vi "Build-temperature-regression.vi"(8 "error in (no error)":errorcluster, 9 "Storage params in":refnum<data-value>, 10 "Acquis. params in":refnum<data-value>, 11 "Temperature params in":refnum<data-value>) -> (0 "error out":errorcluster, 1 "Storage params":refnum<data-value>, 2 "Acquis. params":refnum<data-value>, 3 "Temperature params":refnum<data-value>)   [LabVIEW 2013, in "CameraVision.lvlib" / "CV-Temperature.lvclass"]
uses:
  CV-Temperature.lvclass
  Acquisition/CV-Acquisition.lvclass
  Storage/CV-Storage.lvclass
  Storage/CV-Storage.lvclass/CV-Storage.ctl
  CV-Temperature.lvclass/CV-Temperature.ctl
  Acquisition/CV-Acquisition.lvclass/CV-Acquisition.ctl
  UI/Module-states.ctl
  Write Temperature status.vi
  Write TemperatureFieldRegression.vi
  Acquisition/Read Exposure time camera 1.vi
  Acquisition/Read Exposure time camera 2.vi
  Read Temperature field.vi
  Read Ratio correction factor.vi
  Read Regression file relative path.vi
  Storage/Read Base path.vi
  <vilib>/Utility/file.llb/Read From Spreadsheet File (DBL).vi
  UI/CV-UI.lvclass
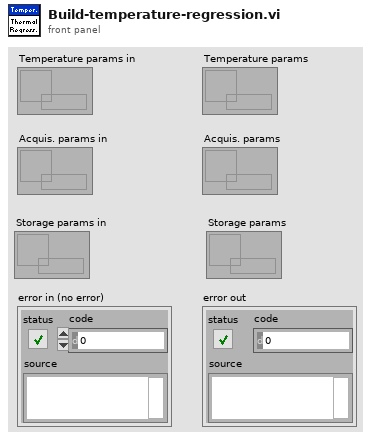
[diagram p1: front panel]
types:
  T1 = typedef "CameraVision.lvlib/CV-UI.lvclass/Module-states.ctl" = enum16{"Inactive", "Active", "Data-loss", "Error", "Simulation", "Synchronizing", "Initialized", "Released"}
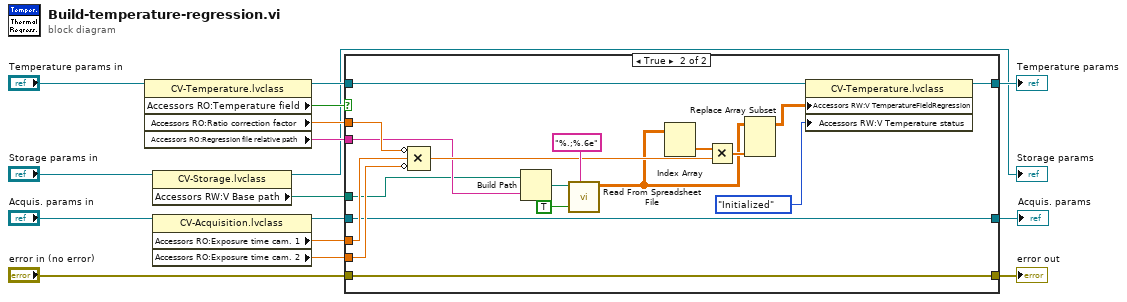
[diagram p0: block diagram]
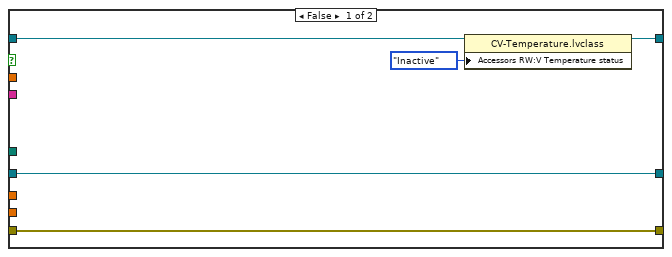
[diagram p2: hidden frame]
diagram:
  n1 = property class="CV-Temperature.lvclass"(reference="Temperature params in") -> (reference out=w9:refnum<data-value>, "Accessors RO:Temperature field"=w8:bool, "Accessors RO:Ratio correction factor"=w7:dbl, "Accessors RO:Regression file relative path"=w10:string)  [unwired: 1 in, 1 out]
  n2 = property class="CV-Storage.lvclass"(reference="Storage params in") -> (reference out=→"Storage params":refnum<data-value>, "Accessors RW:V Base path"=w2:path)  [unwired: 1 in, 1 out]
  n3 = property class="CV-Acquisition.lvclass"(reference="Acquis. params in") -> (reference out=w15:refnum<data-value>, "Accessors RO:Exposure time cam. 1"=w6:dbl, "Accessors RO:Exposure time cam. 2"=w5:dbl)  [unwired: 1 in, 1 out]
  n4 = case shown="True" w8 {
    tunnel: w9 -> [w18 w29]
    tunnel: [w21 w24] -> w4
    tunnel: w5 -> [_ w34]
    tunnel: w6 -> [_ w33]
    tunnel: w7 -> [_ w32]
    tunnel: "error in (no error)" -> [w21 w24]
    tunnel: w10 -> [_ w27]
    tunnel: [w19 w26] -> w14
    tunnel: [w20 w25] -> w16
    tunnel: w15 -> [w20 w25]
    tunnel: w2 -> [_ w22]
    frame False {
      n5 = property class="CV-Temperature.lvclass"(reference=w18, "Accessors RW:V Temperature status"=Module-states."Inactive" ("V Temperature status")) -> (reference out=w19:refnum<data-value>)  [unwired: 1 in, 1 out]
    }
    frame True {
      n6 = Compound Arithmetic op=MULTIPLY(invert w32, w33, invert w34) -> (w31:dbl)
      n7 = Build Path(base path=w22, name or relative path=w27) -> (appended path=w39:path)
      n8 = call-poly <vilib>:"Read From Spreadsheet File.vi"("transpose (no:F)"=TRUE, "format (%.3f)"="%.;%.6e", "file path (dialog if empty)"=w39) -> ("all rows"=w30:dbl[][])  [unwired: 4 in, 4 out]
      n9 = Index Array(array=w30) -> (element=w36:dbl[])  [unwired: 2 in]
      n10 = Multiply(x=w36, y=w31) -> (x*y=w35:dbl[])
      n11 = Replace Array Subset(array=w30, new element=w35) -> (w28:dbl[][])  [unwired: 2 in]
      n12 = property class="CV-Temperature.lvclass"(reference=w29, "Accessors RW:V TemperatureFieldRegression"=w28, "Accessors RW:V Temperature status"=Module-states."Initialized" ("V Temperature status")) -> (reference out=w26:refnum<data-value>)  [unwired: 1 in, 1 out]
    }
  }
  "Acquis. params" <- w16
  "Temperature params" <- w14
  "error out" <- w4
